vi "user output.vi"(8 "error in":errorcluster, 11 "Outputs to system":T1) -> (0 "error out":errorcluster)   [LabVIEW 2013, in "fixed channel tag bus module.lvclass"]
uses:
  fixed channel tag bus module.lvclass
  output user data.ctl
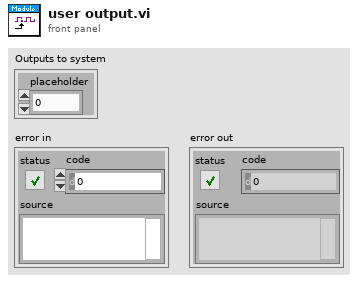
[diagram p1: front panel]
types:
  T1 = typedef "fixed channel tag bus module.lvclass/output user data.ctl" = cluster{"placeholder":sgl}
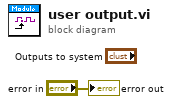
[diagram p0: block diagram]
diagram:
  "error out" <- "error in"
